vi "WILT Search For Valve Channel.vi"(9 "Start Buttons Cluster":T3, 10 "Water Valves Cluster":T2, 11 "Agilent Valve and Switch Locations":T1[](array[typedef])=[{"Channel"="301", "Station"="1", "Label"="Water Valve", "Agilent Station"="2", "Data"=0.0}, {"Channel"="302", "Station"="2", "Label"="Water Valve", "Agilent Station"="2", "Data"=0.0}, {"Channel"="303", "Station"="3", "Label"="Water Valve", "Agilent Station"="2", "Data"=0.0}, {"Channel"="304", "Station"="4", "Label"="Water Valve", "Agilent Station"="2", "Data"=0.0}, {"Channel"="305", "Station"="5", "Label"="Water Valve", "Agilent Station"="2", "Data"=0.0}, {"Channel"="306", "Station"="6", "Label"="Water Valve", "Agilent Station"="2", "Data"=0.0}, {"Channel"="307", "Station"="7", "Label"="Water Valve", "Agilent Station"="2", "Data"=0.0}, {"Channel"="308", "Station"="8", "Label"="Water Valve", "Agilent Station"="2", "Data"=0.0}, {"Channel"="309", "Station"="9", "Label"="Water Valve", "Agilent Station"="2", "Data"=0.0}, {"Channel"="310", "Station"="10", "Label"="Water Valve", "Agilent Station"="2", "Data"=0.0}, {"Channel"="311", "Station"="11", "Label"="Water Valve", "Agilent Station"="2", "Data"=0.0}, {"Channel"="312", "Station"="12", "Label"="Water Valve", "Agilent Station"="2", "Data"=0.0}, {"Channel"="313", "Station"="13", "Label"="Water Valve", "Agilent Station"="2", "Data"=0.0}, {"Channel"="314", "Station"="14", "Label"="Water Valve", "Agilent Station"="2", "Data"=0.0}, {"Channel"="315", "Station"="15", "Label"="Water Valve", "Agilent Station"="2", "Data"=0.0}, {"Channel"="316", "Station"="16", "Label"="Water Valve", "Agilent Station"="2", "Data"=0.0}, {"Channel"="317", "Station"="17", "Label"="Water Valve", "Agilent Station"="2", "Data"=0.0}, {"Channel"="318", "Station"="18", "Label"="Water Valve", "Agilent Station"="2", "Data"=0.0}, {"Channel"="319", "Station"="19", "Label"="Water Valve", "Agilent Station"="2", "Data"=0.0}, {"Channel"="320", "Station"="20", "Label"="Water Valve", "Agilent Station"="2", "Data"=0.0}, {"Channel"="101", "Station"="21", "Label"="Water Valve", "Agilent Station"="3", "Data"=0.0}, {"Channel"="102", "Station"="22", "Label"="Water Valve", "Agilent Station"="3", "Data"=0.0}, {"Channel"="103", "Station"="23", "Label"="Water Valve", "Agilent Station"="3", "Data"=0.0}, {"Channel"="104", "Station"="24", "Label"="Water Valve", "Agilent Station"="3", "Data"=0.0}, {"Channel"="105", "Station"="25", "Label"="Water Valve", "Agilent Station"="3", "Data"=0.0}, {"Channel"="106", "Station"="26", "Label"="Water Valve", "Agilent Station"="3", "Data"=0.0}, {"Channel"="107", "Station"="27", "Label"="Water Valve", "Agilent Station"="3", "Data"=0.0}, {"Channel"="108", "Station"="28", "Label"="Water Valve", "Agilent Station"="3", "Data"=0.0}, {"Channel"="109", "Station"="29", "Label"="Water Valve", "Agilent Station"="3", "Data"=0.0}, {"Channel"="110", "Station"="30", "Label"="Water Valve", "Agilent Station"="3", "Data"=0.0}, {"Channel"="111", "Station"="31", "Label"="Water Valve", "Agilent Station"="3", "Data"=0.0}, {"Channel"="112", "Station"="32", "Label"="Water Valve", "Agilent Station"="3", "Data"=0.0}, {"Channel"="101", "Station"="33", "Label"="Water Valve", "Agilent Station"="5", "Data"=0.0}, {"Channel"="102", "Station"="34", "Label"="Water Valve", "Agilent Station"="5", "Data"=0.0}, {"Channel"="103", "Station"="35", "Label"="Water Valve", "Agilent Station"="5", "Data"=0.0}, {"Channel"="104", "Station"="36", "Label"="Water Valve", "Agilent Station"="5", "Data"=0.0}, {"Channel"="105", "Station"="37", "Label"="Water Valve", "Agilent Station"="5", "Data"=0.0}, {"Channel"="106", "Station"="38", "Label"="Water Valve", "Agilent Station"="5", "Data"=0.0}, {"Channel"="107", "Station"="39", "Label"="Water Valve", "Agilent Station"="5", "Data"=0.0}, {"Channel"="108", "Station"="40", "Label"="Water Valve", "Agilent Station"="5", "Data"=0.0}, {"Channel"="109", "Station"="41", "Label"="Water Valve", "Agilent Station"="5", "Data"=0.0}, {"Channel"="110", "Station"="42", "Label"="Water Valve", "Agilent Station"="5", "Data"=0.0}, {"Channel"="111", "Station"="43", "Label"="Water Valve", "Agilent Station"="5", "Data"=0.0}, {"Channel"="112", "Station"="44", "Label"="Water Valve", "Agilent Station"="5", "Data"=0.0}, {"Channel"="113", "Station"="45", "Label"="Water Valve", "Agilent Station"="5", "Data"=0.0}, {"Channel"="114", "Station"="46", "Label"="Water Valve", "Agilent Station"="5", "Data"=0.0}, {"Channel"="115", "Station"="47", "Label"="Water Valve", "Agilent Station"="5", "Data"=0.0}, {"Channel"="116", "Station"="48", "Label"="Water Valve", "Agilent Station"="5", "Data"=0.0}, {"Channel"="117", "Station"="49", "Label"="Water Valve", "Agilent Station"="5", "Data"=0.0}, {"Channel"="118", "Station"="50", "Label"="Water Valve", "Agilent Station"="5", "Data"=0.0}, {"Channel"="119", "Station"="51", "Label"="Water Valve", "Agilent Station"="5", "Data"=0.0}, {"Channel"="120", "Station"="52", "Label"="Water Valve", "Agilent Station"="5", "Data"=0.0}, {"Channel"="201", "Station"="53", "Label"="Water Valve", "Agilent Station"="5", "Data"=0.0}, {"Channel"="202", "Station"="54", "Label"="Water Valve", "Agilent Station"="5", "Data"=0.0}, {"Channel"="203", "Station"="55", "Label"="Water Valve", "Agilent Station"="5", "Data"=0.0}, {"Channel"="204", "Station"="56", "Label"="Water Valve", "Agilent Station"="5", "Data"=0.0}, {"Channel"="301", "Station"="21", "Label"="Start Button", "Agilent Station"="5", "Data"=0.0}, {"Channel"="302", "Station"="22", "Label"="Start Button", "Agilent Station"="5", "Data"=0.0}, {"Channel"="303", "Station"="23", "Label"="Start Button", "Agilent Station"="5", "Data"=0.0}, {"Channel"="304", "Station"="24", "Label"="Start Button", "Agilent Station"="5", "Data"=0.0}, {"Channel"="305", "Station"="25", "Label"="Start Button", "Agilent Station"="5", "Data"=0.0}, {"Channel"="306", "Station"="26", "Label"="Start Button", "Agilent Station"="5", "Data"=0.0}, {"Channel"="307", "Station"="27", "Label"="Start Button", "Agilent Station"="5", "Data"=0.0}, {"Channel"="308", "Station"="28", "Label"="Start Button", "Agilent Station"="5", "Data"=0.0}, {"Channel"="309", "Station"="29", "Label"="Start Button", "Agilent Station"="5", "Data"=0.0}, {"Channel"="310", "Station"="30", "Label"="Start Button", "Agilent Station"="5", "Data"=0.0}, {"Channel"="311", "Station"="31", "Label"="Start Button", "Agilent Station"="5", "Data"=0.0}, {"Channel"="312", "Station"="32", "Label"="Start Button", "Agilent Station"="5", "Data"=0.0}, {"Channel"="101", "Station"="33", "Label"="Start Button", "Agilent Station"="7", "Data"=0.0}, {"Channel"="102", "Station"="34", "Label"="Start Button", "Agilent Station"="7", "Data"=0.0}, {"Channel"="103", "Station"="35", "Label"="Start Button", "Agilent Station"="7", "Data"=0.0}, {"Channel"="104", "Station"="36", "Label"="Start Button", "Agilent Station"="7", "Data"=0.0}, {"Channel"="105", "Station"="37", "Label"="Start Button", "Agilent Station"="7", "Data"=0.0}, {"Channel"="106", "Station"="38", "Label"="Start Button", "Agilent Station"="7", "Data"=0.0}, {"Channel"="107", "Station"="39", "Label"="Start Button", "Agilent Station"="7", "Data"=0.0}, {"Channel"="108", "Station"="40", "Label"="Start Button", "Agilent Station"="7", "Data"=0.0}, {"Channel"="109", "Station"="41", "Label"="Start Button", "Agilent Station"="7", "Data"=0.0}, {"Channel"="110", "Station"="42", "Label"="Start Button", "Agilent Station"="7", "Data"=0.0}, {"Channel"="111", "Station"="43", "Label"="Start Button", "Agilent Station"="7", "Data"=0.0}, {"Channel"="112", "Station"="44", "Label"="Start Button", "Agilent Station"="7", "Data"=0.0}]) -> (0 "Station Number":string, 1 "Channel":string, 2 "Agilent Station":string, 3 "Label":string)   [LabVIEW 2016]
uses:
  Type Definitions/WILT Start Button Cluster.ctl
  Type Definitions/WILT Water Valve Cluster.ctl
  Type Definitions/WILT Agilent Channel Definition.ctl
  <vilib>/Utility/error.llb/whitespace.ctl
panel:
  out "Start Button Array":bool[](array[boolean])
  out "Water Valve Array":bool[](array[boolean])
  out "Label (Water Valve)":string
  out "Label (Start Button)":string
  out "Channel Start Button":string
  out "Agilent Station Start Button":string
  out "Agilent Station Water Valve":string
  out "Channel Water Valve":string
  out "Water Valve Station Number":i32
  out "Station Number Start Button":i32
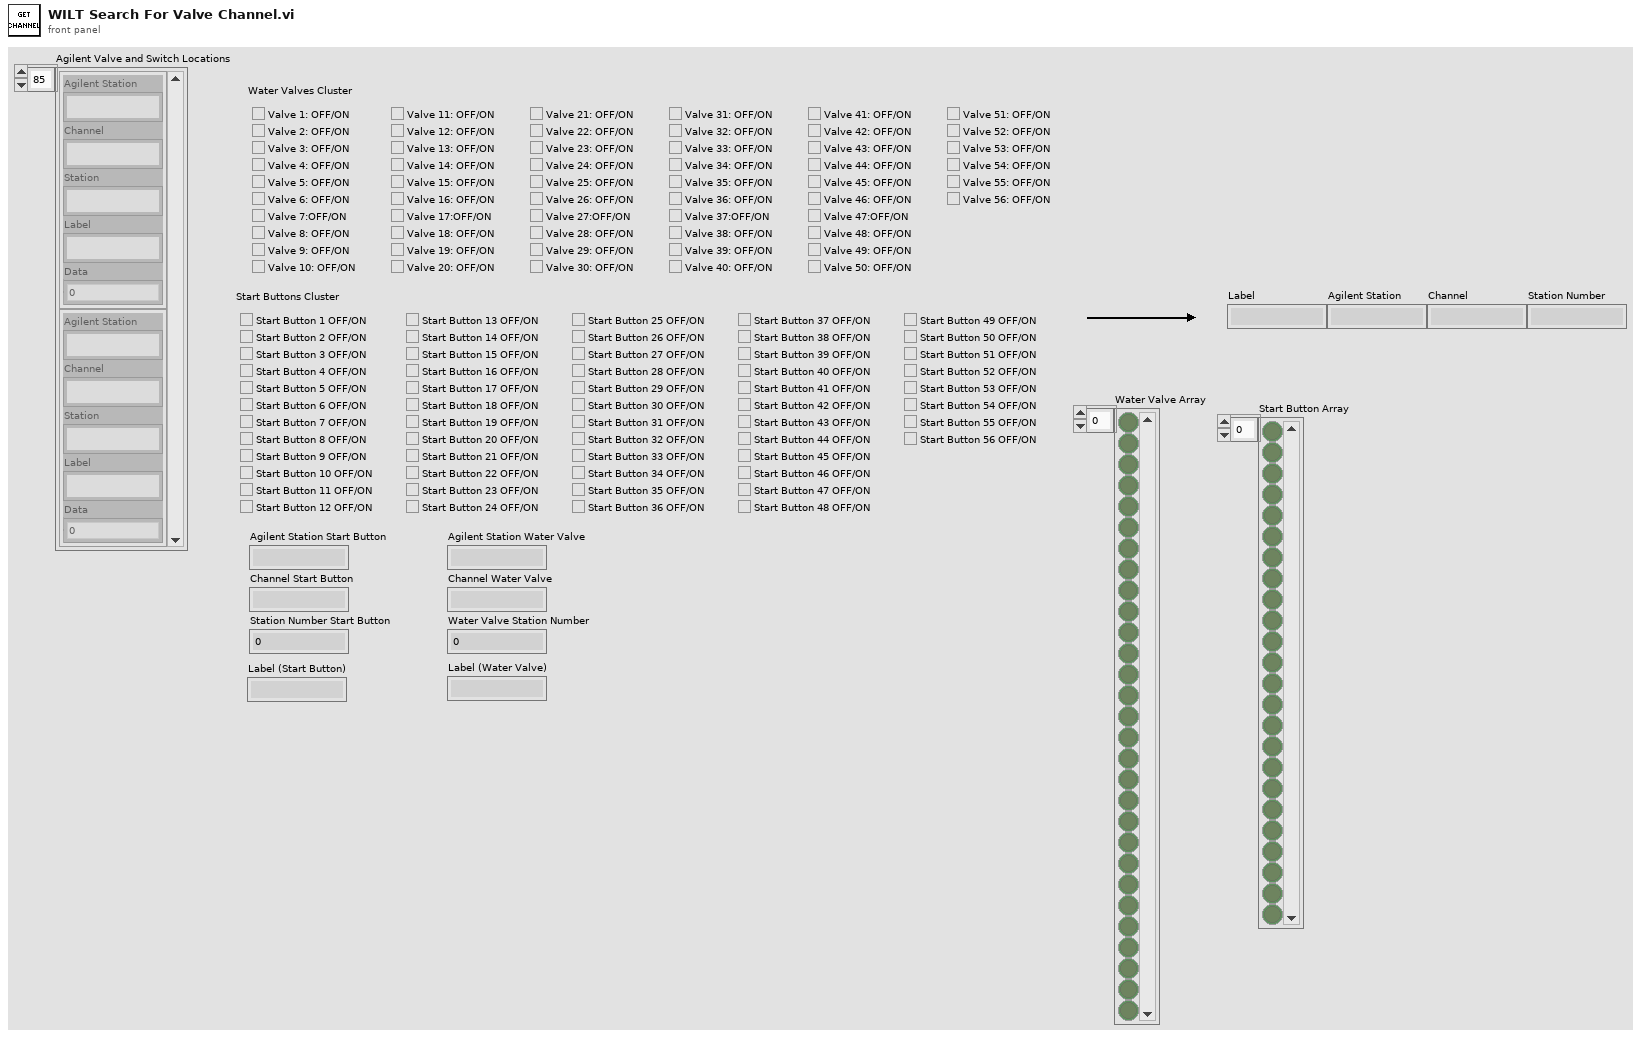
[diagram p1: front panel]
types:
  T1 = typedef "WILT Agilent Channel Definition.ctl" = cluster{"Channel":string, "Station":string, "Label":string, "Agilent Station":string, "Data":dbl}
  T2 = typedef "WILT Water Valve Cluster.ctl" = cluster{"Valve 1":bool, "Valve 2":bool, "Valve 3":bool, "Valve 4":bool, "Valve 5":bool, "Valve 6":bool, "Valve 7":bool, "Valve 8":bool, "Valve 9":bool, "Valve 10":bool, "Valve 11":bool, "Valve 12":bool, "Valve 13":bool, "Valve 14":bool, "Valve 15":bool, "Valve 16":bool, "Valve 17":bool, "Valve 18":bool, "Valve 19":bool, "Valve 20":bool, "Valve 21":bool, "Valve 22":bool, "Valve 23":bool, "Valve 24":bool, "Valve 25":bool, "Valve 26":bool, "Valve 27":bool, "Valve 28":bool, "Valve 29":bool, "Valve 30":bool, "Valve 31":bool, "Valve 32":bool, "Valve 33":bool, "Valve 34":bool, "Valve 35":bool, "Valve 36":bool, "Valve 37":bool, "Valve 38":bool, "Valve 39":bool, "Valve 40":bool, "Valve 41":bool, "Valve 42":bool, "Valve 43":bool, "Valve 44":bool, "Valve 45":bool, "Valve 46":bool, "Valve 47":bool, "Valve 48":bool, "Valve 49":bool, "Valve 50":bool, "Valve 51":bool, "Valve 52":bool, "Valve 53":bool, "Valve 54":bool, "Valve 55":bool, "Valve 56":bool}
  T3 = typedef "WILT Start Button Cluster.ctl" = cluster{"Start Button 21":bool, "Start Button 22":bool, "Start Button 23":bool, "Start Button 24":bool, "Start Button 25":bool, "Start Button 26":bool, "Start Button 27":bool, "Start Button 28":bool, "Start Button 29":bool, "Start Button 30":bool, "Start Button 31":bool, "Start Button 32":bool, "Start Button 33":bool, "Start Button 34":bool, "Start Button 35":bool, "Start Button 36":bool, "Start Button 37":bool, "Start Button 38":bool, "Start Button 39":bool, "Start Button 40":bool, "Start Button 41":bool, "Start Button 42":bool, "Start Button 43":bool, "Start Button 44":bool, "Start Button 12":bool, "Start Button 11":bool, "Start Button 10":bool, "Start Button 9":bool, "Start Button 8":bool, "Start Button 7":bool, "Start Button 6":bool, "Start Button 5":bool, "Start Button 4":bool, "Start Button 3":bool, "Start Button 2":bool, "Start Button 1":bool, "Start Button 20":bool, "Start Button 19":bool, "Start Button 18":bool, "Start Button 17":bool, "Start Button 16":bool, "Start Button 15":bool, "Start Button 14":bool, "Start Button 13":bool, "Start Button 45":bool, "Start Button 46":bool, "Start Button 47":bool, "Start Button 48":bool, "Start Button 49":bool, "Start Button 50":bool, "Start Button 51":bool, "Start Button 52":bool, "Start Button 53":bool, "Start Button 54":bool, "Start Button 55":bool, "Start Button 56":bool}
  T4 = typedef "whitespace.ctl" = u16
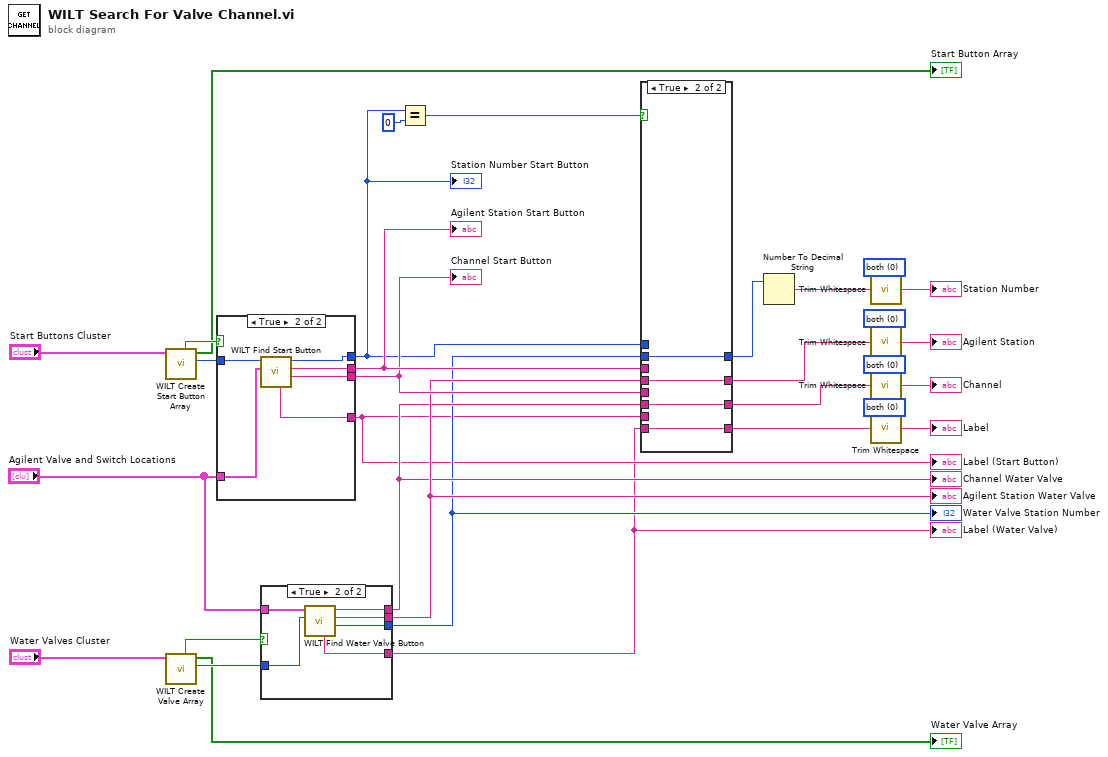
[diagram p0: block diagram]
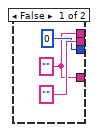
[diagram p3: hidden frame]
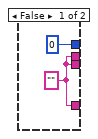
[diagram p4: hidden frame]
diagram:
  w5 = T4 0 items=["both", "start of string", "end of string"] ("location (both)")
  w8 = T4 0 items=["both", "start of string", "end of string"] ("location (both)")
  w11 = T4 0 items=["both", "start of string", "end of string"] ("location (both)")
  w14 = T4 0 items=["both", "start of string", "end of string"] ("location (both)")
  n1 = call "WILT Create Start Button Array.vi"("Start Buttons Cluster"="Start Buttons Cluster") -> ("Station Number"=w28:i32, "Start Button Array"=→"Start Button Array":bool[], "Valve Found!!"=w27:bool)  [unwired: 8 in]
  n2 = call "WILT Create Valve Array.vi"("Water Valves Cluster"="Water Valves Cluster") -> ("Station Number"=w30:i32, "Water Valve Array"=→"Water Valve Array":bool[], "Valve Found!!"=w26:bool)  [unwired: 8 in]
  n3 = case shown="True" w27 {
    tunnel: "Agilent Valve and Switch Locations" -> [_ w40]
    tunnel: w28 -> [_ w39]
    tunnel: [w33 w38] -> w23
    tunnel: [w33 w37] -> w22
    tunnel: [0 w36] -> w21
    tunnel: [w33 w35] -> w16
    frame False {
      w33 = "" ("Agilent Station")
    }
    frame True {
      n4 = call "WILT Find Start Button.vi"("Agilent Valve and Switch Locations"=w40, "Station Number"=w39) -> ("Channel"=w37:string, "Agilent Station"=w38:string, "Station Number"=w36:i32, "Label"=w35:string)  [unwired: 6 in]
    }
  }
  "Station Number Start Button" <- w21
  "Agilent Station Start Button" <- w23
  "Channel Start Button" <- w22
  "Label (Start Button)" <- w16
  n5 = case shown="True" w26 {
    tunnel: w30 -> [_ w49]
    tunnel: [w41 w48] -> w19
    tunnel: ["" ("Agilent Station") w47] -> w20
    tunnel: "Agilent Valve and Switch Locations" -> [_ w46]
    tunnel: [0 w45] -> w18
    tunnel: [w41 w44] -> w15
    frame False {
      w41 = "" ("Channel")
    }
    frame True {
      n6 = call "WILT Find Water Valve Button.vi"("Station Number"=w49, "Agilent Valve and Switch Locations"=w46) -> ("Station Number"=w45:i32, "Agilent Station"=w47:string, "Channel"=w48:string, "Label"=w44:string)  [unwired: 5 in, 1 out]
    }
  }
  "Water Valve Station Number" <- w18
  "Channel Water Valve" <- w19
  "Agilent Station Water Valve" <- w20
  "Label (Water Valve)" <- w15
  n7 = Equal?(x=w21, y=0) -> (x = y?=w24:bool)
  n8 = case shown="True" w24 {
    tunnel: w18 -> [_ w55]
    tunnel: w19 -> [_ w56]
    tunnel: w20 -> [_ w57]
    tunnel: [w53 w57] -> w13
    tunnel: [w52 w56] -> w10
    tunnel: [w51 w55] -> w17
    tunnel: w23 -> [w53 _]
    tunnel: w22 -> [w52 _]
    tunnel: w21 -> [w51 _]
    tunnel: w16 -> [w50 _]
    tunnel: [w50 w54] -> w4
    tunnel: w15 -> [_ w54]
    frame False {
    }
    frame True {
    }
  }
  n9 = Number To Decimal String(number=w17) -> (decimal integer string=w7:string)  [unwired: 1 in]
  n10 = call <vilib>:"Trim Whitespace.vi"("string"=w7, "location (both)"=w8) -> ("trimmed string"=→"Station Number":string)
  n11 = call <vilib>:"Trim Whitespace.vi"("string"=w13, "location (both)"=w14) -> ("trimmed string"=→"Agilent Station":string)
  n12 = call <vilib>:"Trim Whitespace.vi"("string"=w10, "location (both)"=w11) -> ("trimmed string"=→"Channel":string)
  n13 = call <vilib>:"Trim Whitespace.vi"("string"=w4, "location (both)"=w5) -> ("trimmed string"=→"Label":string)
